vi "Configure Limit Test Comparison.vi"(6 "Enable Save Waveform (False)":bool, 7 "Template Waveform (0:Reference Waveform 1)":i32(ring) items=["Reference Waveform 1", "Reference Waveform 2", "Reference Waveform 3", "Reference Waveform 4"], 8 "error in (no error)":errorcluster, 9 "Enable Save Image (False)":bool, 10 "Source (0:Channel 1)":i32(ring) items=["Channel 1", "Channel 2", "Channel 3", "Channel 4", "Math"], 11 "VISA resource name":refnum<visa-resource-name>) -> (0 "error out":errorcluster, 3 "VISA resource name out":refnum<visa-resource-name>)   [LabVIEW 2017, in "Tektronix TDS 200 1000 2000 Series.lvlib"]
doc: "This VI configures the settings for a limit test comparison.\n\n<b>Note(s):</b>\nThis VI does not check the instrument status."
uses:
  Tektronix TDS 200 1000 2000 Series.lvlib
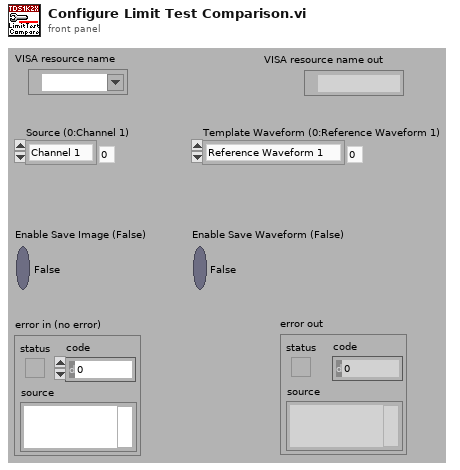
[diagram p1: front panel]
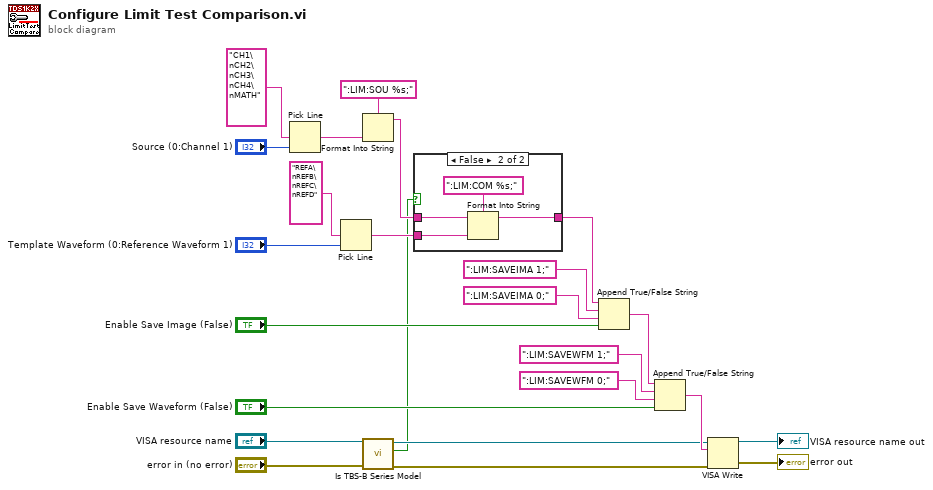
[diagram p0: block diagram]
diagram:
  n1 = Pick Line(multi-line string="CH1\nCH2\nCH3\nCH4\nMATH", line index="Source (0:Channel 1)") -> (output string=w16:string)  [unwired: 1 out]
  n2 = Pick Line(multi-line string="REFA\nREFB\nREFC\nREFD", line index="Template Waveform (0:Reference Waveform 1)") -> (output string=w6:string)  [unwired: 1 out]
  n3 = Format Into String(format string=":LIM:SOU %s;", w16) -> (resulting string=w12:string)  [unwired: 2 in, 1 out]
  n4 = call "Is TBS-B Series Model.vi"("error in (no error)"="error in (no error)", "VISA resource name"="VISA resource name") -> ("error out"=w2:errorcluster, "Is TBS-B Series Model"=w1:bool, "VISA resource name out"=w3:refnum<visa-resource-name>)  [unwired: 7 out]
  n5 = case shown="False" w1 {
    tunnel: [w25 w28] -> w13
    tunnel: w12 -> [w25 w27]
    tunnel: w6 -> [_ w26]
    frame True {
      # "TBS-B Series models"
    }
    frame False {
      n6 = Format Into String(format string=":LIM:COM %s;", initial string=w27, w26) -> (resulting string=w28:string)  [unwired: 1 in, 1 out]
    }
  }
  n7 = Append True/False String(1:"Enable Save Image (False)", 2:":LIM:SAVEIMA 0;", 3:":LIM:SAVEIMA 1;", 4:w13) -> (0:w15:string)
  n8 = Append True/False String(1:"Enable Save Waveform (False)", 2:":LIM:SAVEWFM 0;", 3:":LIM:SAVEWFM 1;", 4:w15) -> (0:w14:string)
  n9 = VISA Write(VISA resource name=w3, write buffer=w14, error in (no error)=w2) -> (VISA resource name out=→"VISA resource name out":refnum<visa-resource-name>, error out=→"error out":errorcluster)  [unwired: 1 out]
